vi "Process.vi"(8 "error in (no error)":errorcluster, 11 "SMO.UI":refnum<class "SMO.UI.Template.lvclass">) -> (0 "error out":errorcluster, 3 "SMO.UI out":refnum<class "SMO.UI.Template.lvclass">)   [LabVIEW 2013, in "SMO.UI.Template.lvclass"]
uses:
  SMO.UI.Template.lvclass
  SMO/Typedefs/Parent Call--Enum.ctl
  SMO.UI/SMO.UI.lvclass
  SMO.UI.Template.lvclass/SMO.UI.Template.ctl
  SMO.Template/SMO.Template.lvclass
  SMO/SMO.lvclass
panel:
  in  "OK":bool
  in  "Set Data":bool
  in  "New Data":string
  out "Data":string
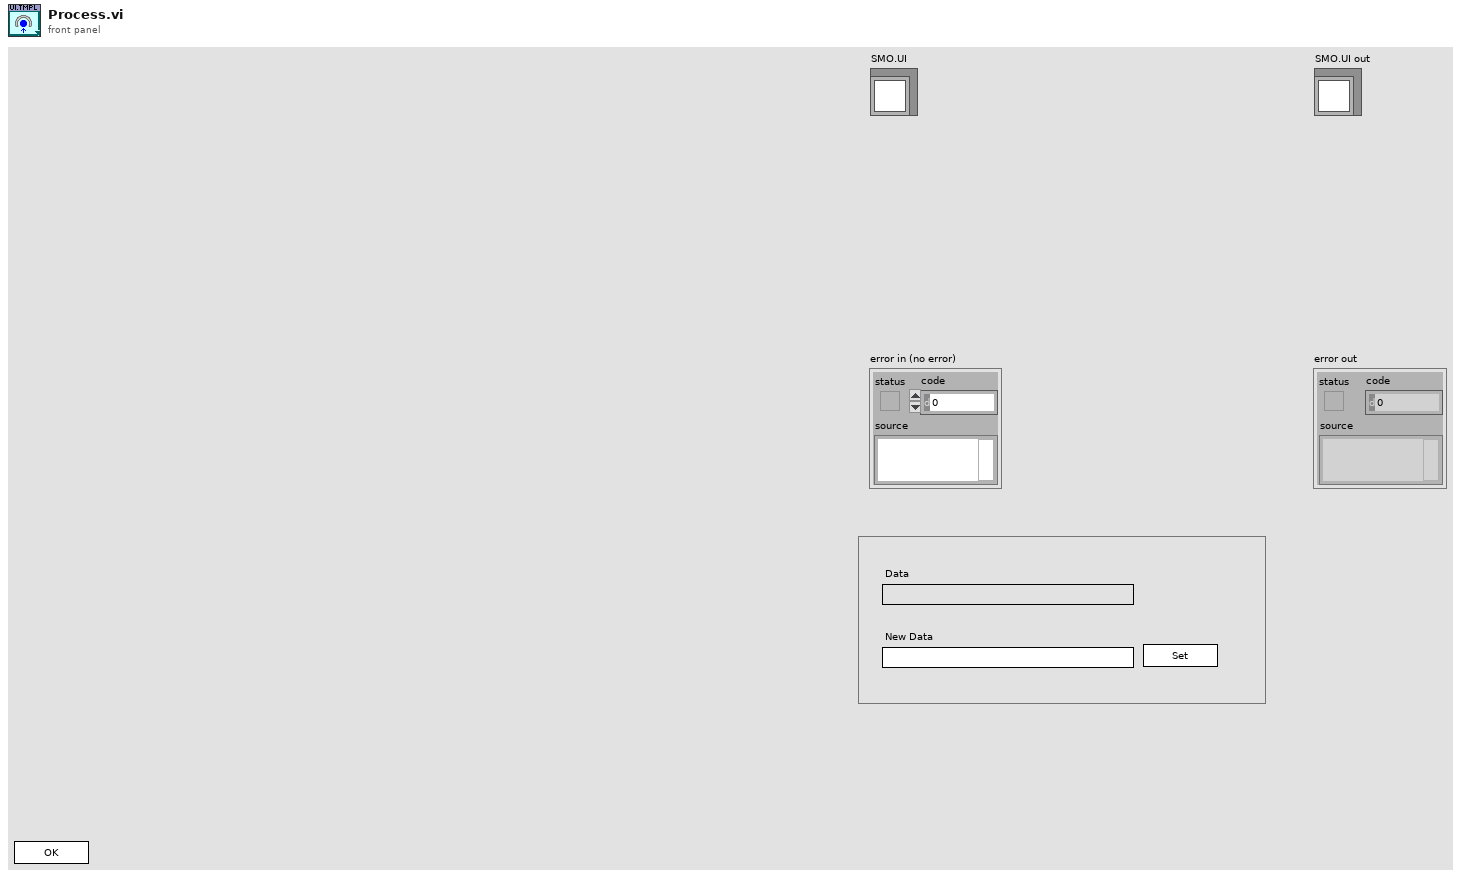
[diagram p1: front panel]
types:
  T1 = typedef "SMO.lvclass/Parent Call--Enum.ctl" = enum16{"Allows parent to run", "Does not request parent to run"}
  T2 = enum32{"invalid app kind", "Development System", "Run Time System", "Student Edition", "Embedded LabVIEW", "Evaluation", "Custom"}
  T3 = enum32{"Invalid", "Standard", "Closed", "Hidden", "Minimized", "Maximized"}
  T4 = cluster{"Core":cluster{"Current VI Reference":refnum<vi>, "Close Panel on Exit?":bool, "error":errorcluster}, "Self Ref":refnum<class "SMO.UI.Template.lvclass">, "Exec.State":enum32{"Bad", "Idle", "Run top level", "Running"}, "SMO.Template":refnum<class "SMO.Template.lvclass">}
  T5 = cluster{"Current VI Reference":refnum<vi>, "Close Panel on Exit?":bool, "error":errorcluster}
  T6 = enum32{"Bad", "Idle", "Run top level", "Running"}
  T7 = typedef "SMO.lvclass/Protected Events.ctl" = cluster{"StopProcesses":refnum<user-event>, "AbortProcesses":refnum<user-event>}
  T8 = cluster{"Event Registration Refnum":refnum<event-registration>, "SMO.UI Public Events":refnum<event-registration>, "SMO.Template Public Events":refnum<event-registration>}
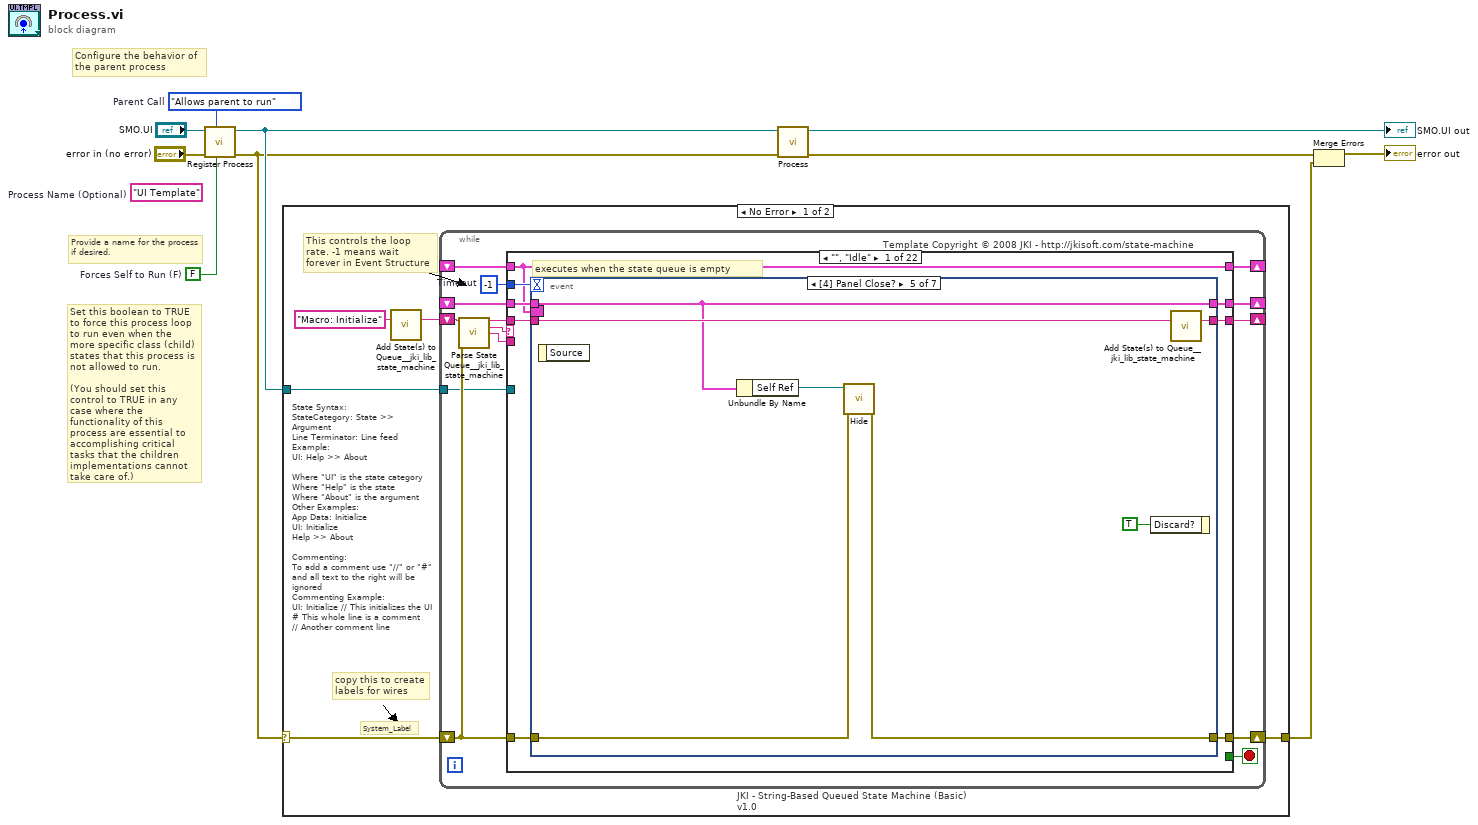
[diagram p0: block diagram]
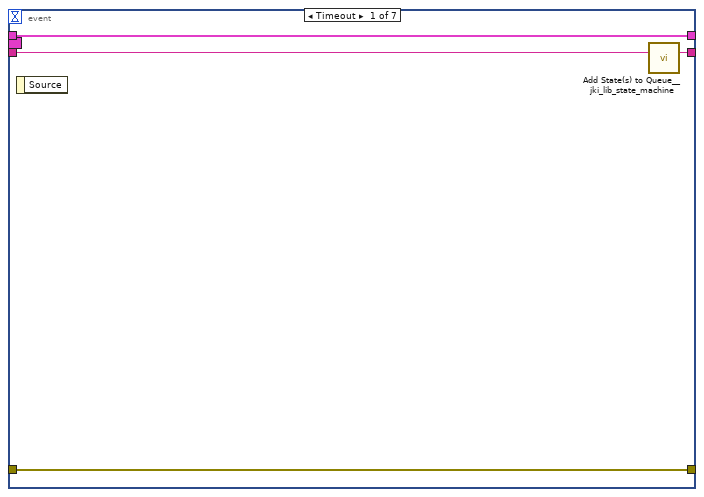
[diagram p2: hidden frame]
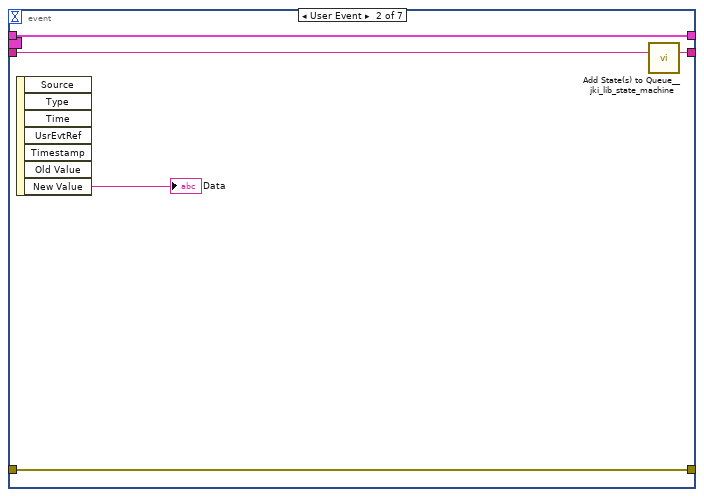
[diagram p3: hidden frame]
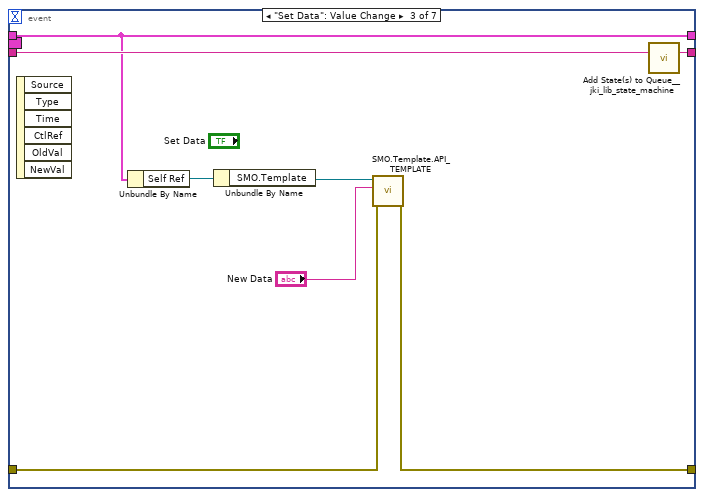
[diagram p4: hidden frame]
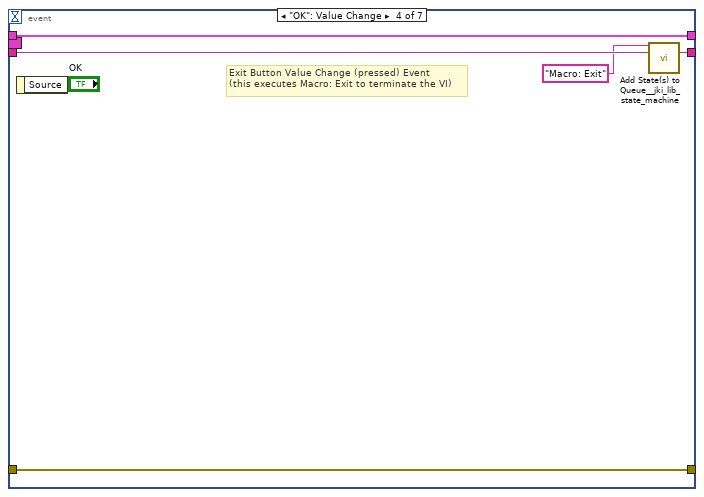
[diagram p5: hidden frame]
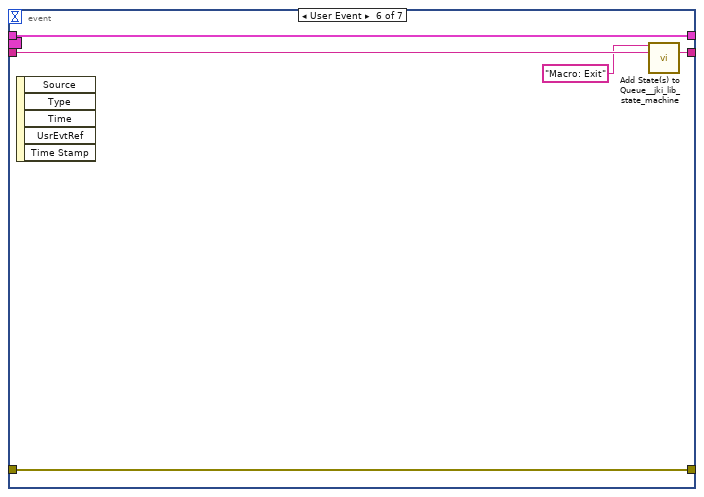
[diagram p6: hidden frame]
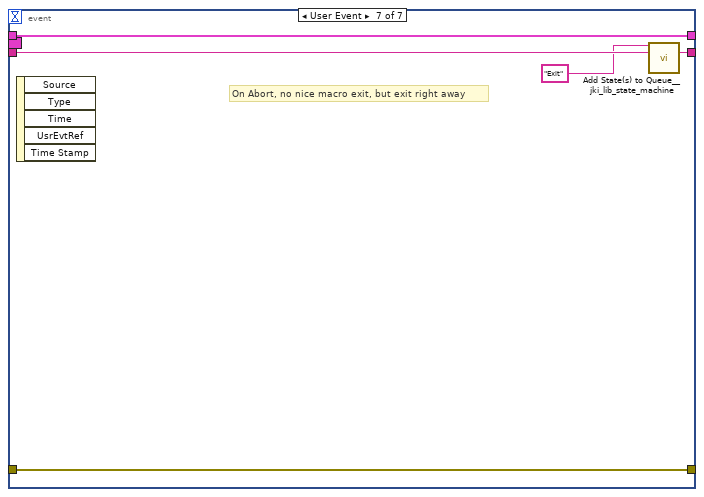
[diagram p7: hidden frame]
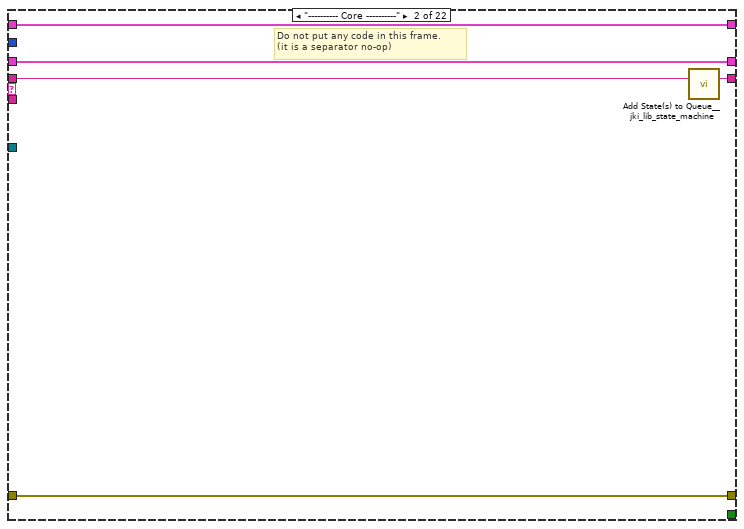
[diagram p8: hidden frame]
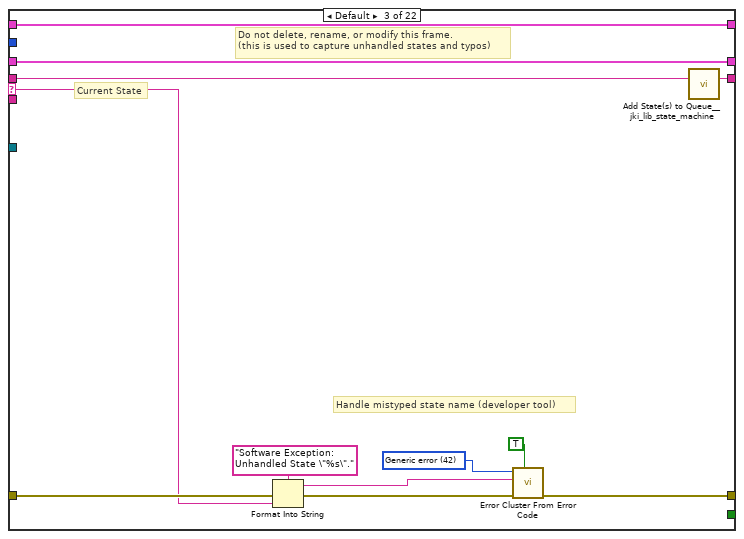
[diagram p9: hidden frame]
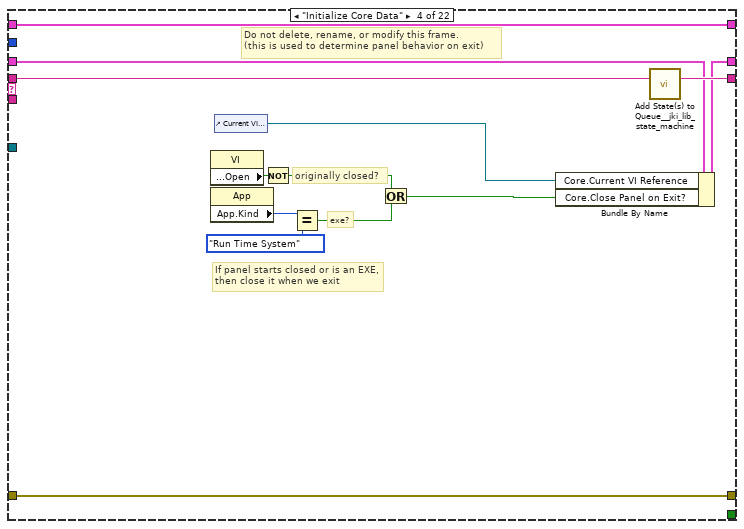
[diagram p10: hidden frame]
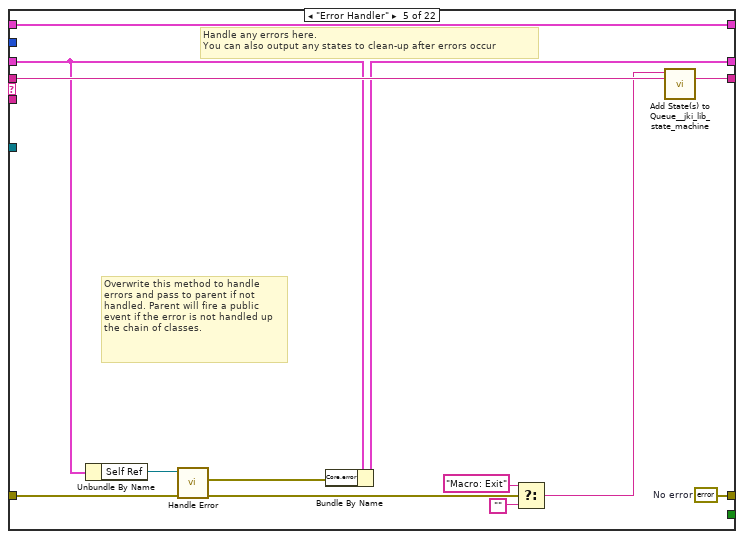
[diagram p11: hidden frame]
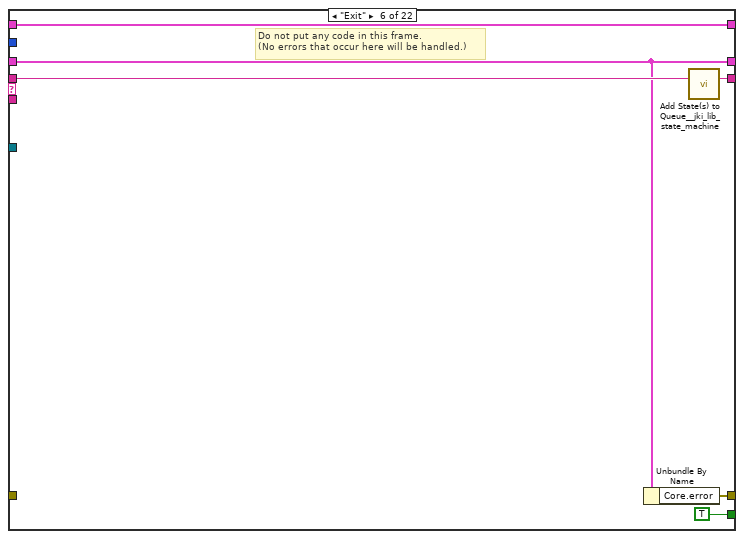
[diagram p12: hidden frame]
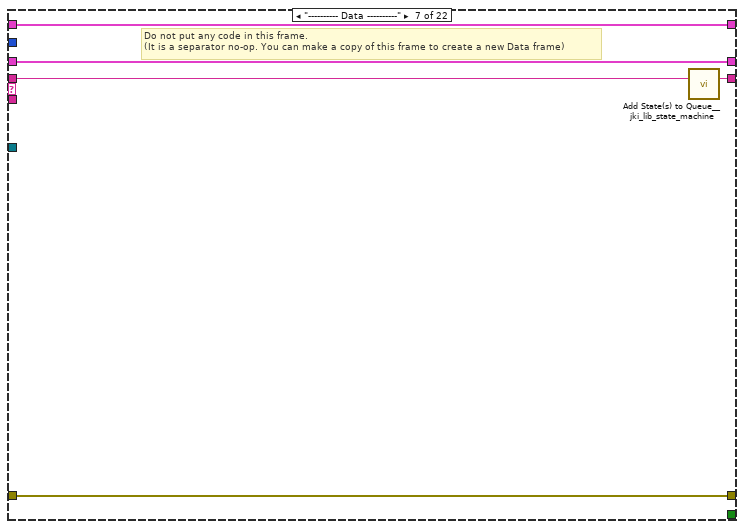
[diagram p13: hidden frame]
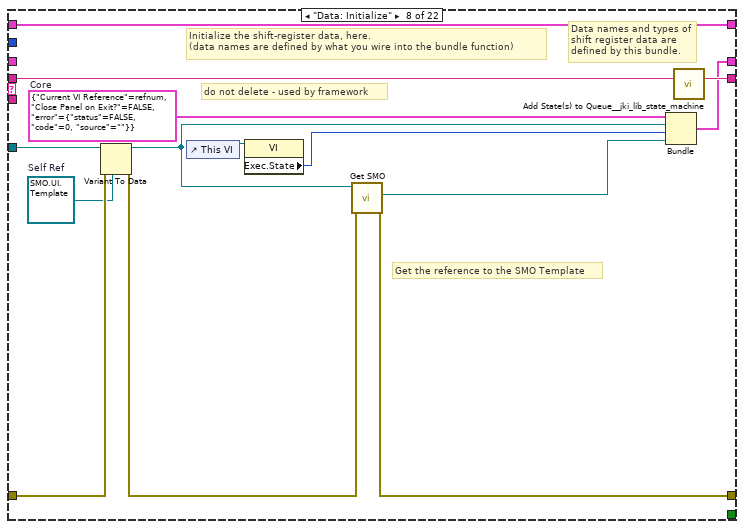
[diagram p14: hidden frame]
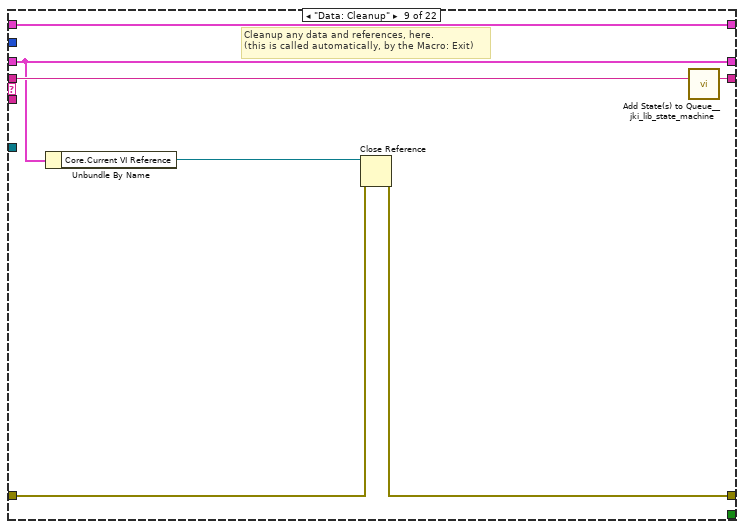
[diagram p15: hidden frame]
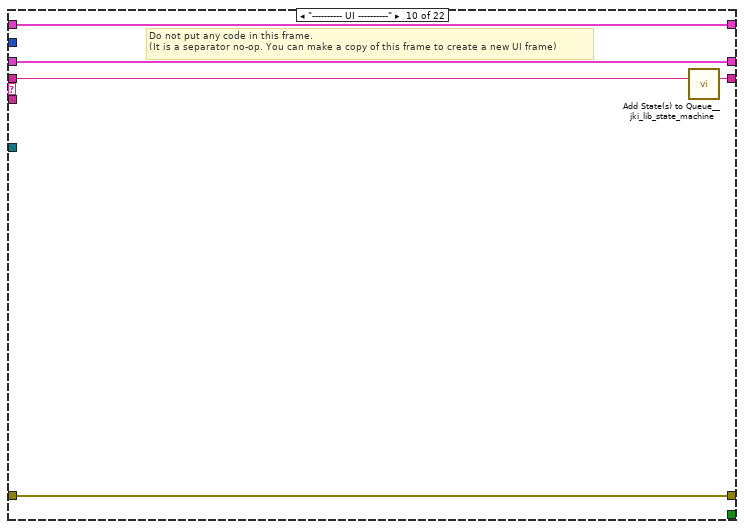
[diagram p16: hidden frame]
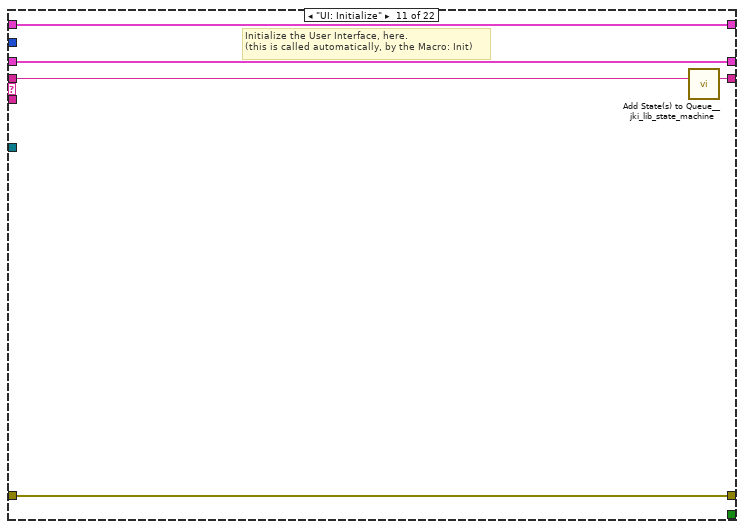
[diagram p17: hidden frame]
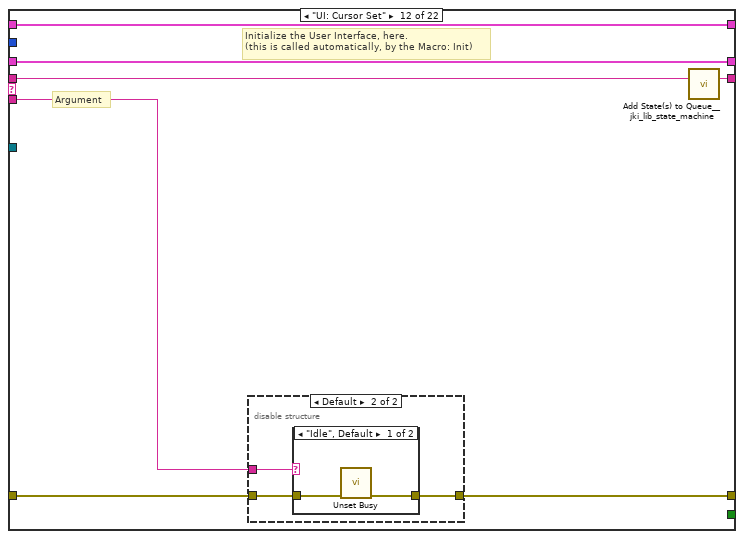
[diagram p18: hidden frame]
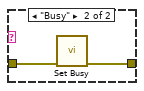
[diagram p20: hidden frame]
diagram:
  w1 = FALSE  # Forces Self to Run (F)
  w2 = Parent_Call--Enum."Allows parent to run"  # Parent Call
  (unwired) "UI Template"  # Process Name (Optional)
  # "Configure the behavior of the parent process"
  # "Provide a name for the process\nif desired."
  # "Set this boolean to TRUE to force this process loop to run even when the more specific class (child) states that this process is not allowed to run.\n\n(You should set this control to TRUE in any case where the functionality of this process are essential to accomplishing critical tasks that the children implementations cannot take care of.)"
  n1 = call "Register Process.vi"("Forces Self to Run (F)"=w1, "Parent Call"=w2, "error in (no error)"="error in (no error)", "SMO"="SMO.UI") -> ("error out"=w4:errorcluster, "SMO out"=w5:refnum<class "SMO.UI.Template.lvclass">)  [unwired: 6 in]
  n2 = case shown="No Error" w4 {
    selector: w4 -> [w12 w294]
    tunnel: w5 -> [w13 _]
    tunnel: [w11 w294] -> w3
    frame No Error {
      # "State Syntax:\nStateCategory: State >> Argument\nLine Terminator: Line feed\nExample:\nUI: Help >> About\n\nWhere \"UI\" is the state category\nWhere \"Help\" is the state\nWhere \"About\" is the argument\nOther Examples:\nApp Data: Initialize\nUI: Initialize\nHelp >> About\n\nCommenting:\nTo add a comment use \"//\" or \"#\" and all text to the right will be ignored\nCommenting Example:\nUI: Initialize // This initializes the UI\n# This whole line is a comment\n// Another comment line"
      # "copy this to create labels for wires"
      # "This controls the loop rate. -1 means wait forever in Event Structure"
      # "System_Label"
      n3 = call <vilib>:"Add State(s) to Queue__jki_lib_state_machine.vi"("State(s) in (\"\")"="Macro: Initialize") -> ("States Out"=w15:string)  [unwired: 14 in]
      n4 = while "JKI - String-Based Queued State Machine (Basic) v1.0" {
        shift-right: [w22] -> _
        shift-left: _ -> [w21]
        shift-right: [w25] -> w11
        shift-left: w12 -> [w19]
        shift-right: [w24] -> _
        shift-left: w15 -> [w26]
        tunnel: w13 -> [w18]
        shift-right: [w17] -> _
        shift-left: _ -> [w16]
        stop <- w23 stop-if-true
        w20 = -1  # Timeout
        # "Template Copyright © 2008 JKI - http://jkisoft.com/state-machine"
        n5 = call <vilib>:"Parse State Queue__jki_lib_state_machine.vi"("State Queue"=w26, "Error In (no error)"=w19) -> ("Remaining States"=w28:string, "Current State"=w29:string, "Arguments"=w27:string)  [unwired: 11 in]
        n6 = case shown="\"\", \"Idle\"" w29 {
          selector: w29 -> [_ _ w83 _ _ _ _ _ _ _ _ _ _ _ _ _ _ _ _ _ _ _]
          tunnel: w28 -> [w37 w81 w87 w106 w119 w125 w130 w144 w151 w156 w161 w168 w184 w216 w225 w239 w244 w255 w265 w282 w288 w293]
          tunnel: w27 -> [_ _ _ _ _ _ _ _ _ _ _ w162 w178 _ _ _ _ _ _ _ _ _]
          tunnel: w21 -> [w35 w78 w85 w97 w110 w121 w127 _ w146 w153 w159 w166 w180 w213 w221 w230 w241 w251 w262 w280 w286 w290]
          tunnel: [w34 w79 w89 w103 w107 w120 w128 w132 w147 w154 w158 w163 w181 w214 w223 w237 w242 w252 w263 w266 w283 w291] -> w25
          tunnel: w19 -> [w33 w79 w88 w103 w111 _ w128 w141 w148 w154 w158 w164 w182 w214 w223 w237 w242 w248 w263 w271 w284 w291]
          tunnel: [w36 w80 w86 w105 w118 w124 w129 w143 w150 w155 w160 w167 w183 w215 w224 w238 w243 w254 w264 w281 w287 w292] -> w24
          tunnel: [_ _ _ _ _ TRUE _ _ _ _ _ _ _ _ _ _ _ _ _ _ _ _] -> w23
          tunnel: [w32 w78 w85 w104 w109 w121 w127 w142 w146 w153 w159 w166 w180 w213 w221 w230 w241 w251 w262 w280 w286 w290] -> w22
          tunnel: w20 -> [w31 _ _ _ _ _ _ _ _ _ _ _ _ _ _ _ _ _ _ _ _ _]
          tunnel: w18 -> [_ _ _ _ _ _ _ w140 _ _ _ _ _ _ _ _ _ _ _ _ _ _]
          tunnel: [w30 w77 w82 w94 w117 w122 w126 w139 w145 w152 w157 w165 w177 w212 w222 w231 w240 w253 w261 w274 w285 w289] -> w17
          tunnel: w16 -> [w30 w77 w82 w94 w117 w122 w126 w139 w145 w152 w157 w165 w177 w212 w222 w231 w240 w253 w261 _ w285 w289]
          frame "", "Idle" {
            # "executes when the state queue is empty"
            n7 = event shown="[4] Panel Close?" {
              selector: w30 -> [_ _ _ _ _ _ _]
              dyn-events: _ -> [_ _ _ _ _ _ _]
              timeout: w31 -> [_ _ _ _ _ _ _]
              tunnel: w37 -> [w41 w46 w54 w59 w66 w71 w76]
              tunnel: [w40 w45 w53 w58 w65 w70 w75] -> w36
              tunnel: w35 -> [w38 w43 w49 w56 w63 w68 w73]
              tunnel: [w39 w44 w47 w57 w60 w69 w74] -> w34
              tunnel: w33 -> [w39 w44 w48 w57 w61 w69 w74]
              tunnel: [w38 w43 w49 w56 w63 w68 w73] -> w32
              event Timeout {
                n8 = event-data() -> ()  [unwired: 1 in, 1 out]
                n9 = call <vilib>:"Add State(s) to Queue__jki_lib_state_machine.vi"("State(s) in (\"\")"=w41) -> ("States Out"=w40:string)  [unwired: 14 in]
              }
              event User Event {
                n10 = event-data() -> ("New Value"=→"Data":string)  [unwired: 1 in, 6 out]
                n11 = call <vilib>:"Add State(s) to Queue__jki_lib_state_machine.vi"("State(s) in (\"\")"=w46) -> ("States Out"=w45:string)  [unwired: 14 in]
              }
              event "Set Data": Value Change {
                n12 = event-data() -> ()  [unwired: 1 in, 6 out]
                n13 = Unbundle By Name(w49) -> ("Self Ref"=w52:refnum<class "SMO.UI.Template.lvclass">)
                n14 = Unbundle By Name(w52) -> ("SMO.Template"=w51:refnum<class "SMO.Template.lvclass">)
                n15 = call "SMO.Template.API_TEMPLATE.vi"("error in (no error)"=w48, "myData"="New Data", "SMO"=w51) -> ("error out"=w47:errorcluster)  [unwired: 6 in, 2 out]
                n16 = call <vilib>:"Add State(s) to Queue__jki_lib_state_machine.vi"("State(s) in (\"\")"=w54) -> ("States Out"=w53:string)  [unwired: 14 in]
              }
              event "OK": Value Change {
                # "Exit Button Value Change (pressed) Event\n(this executes Macro: Exit to terminate the VI)"
                n17 = event-data() -> ()  [unwired: 1 in, 1 out]
                n18 = call <vilib>:"Add State(s) to Queue__jki_lib_state_machine.vi"("State(s) in Front (\"\")"="Macro: Exit", "State(s) in (\"\")"=w59) -> ("States Out"=w58:string)  [unwired: 13 in]
              }
              event Panel Close? {
                n19 = event-data() -> ()  [unwired: 1 in, 1 out]
                n20 = Unbundle By Name(w63) -> ("Self Ref"=w62:refnum<class "SMO.UI.Template.lvclass">)
                n21 = call "Hide.vi"("error in (no error)"=w61, "SMO.UI"=w62) -> ("error out"=w60:errorcluster)  [unwired: 8 in, 1 out]
                n22 = event-data("Discard?"=TRUE) -> ()  [unwired: 1 in, 1 out]
                n23 = call <vilib>:"Add State(s) to Queue__jki_lib_state_machine.vi"("State(s) in (\"\")"=w66) -> ("States Out"=w65:string)  [unwired: 14 in]
              }
              event User Event {
                n24 = event-data() -> ()  [unwired: 1 in, 5 out]
                n25 = call <vilib>:"Add State(s) to Queue__jki_lib_state_machine.vi"("State(s) in Front (\"\")"="Macro: Exit", "State(s) in (\"\")"=w71) -> ("States Out"=w70:string)  [unwired: 13 in]
              }
              event User Event {
                # "On Abort, no nice macro exit, but exit right away"
                n26 = event-data() -> ()  [unwired: 1 in, 5 out]
                n27 = call <vilib>:"Add State(s) to Queue__jki_lib_state_machine.vi"("State(s) in Front (\"\")"="Exit", "State(s) in (\"\")"=w76) -> ("States Out"=w75:string)  [unwired: 13 in]
              }
            }
          }
          frame "---------- Core ----------" {
            # "Do not put any code in this frame.\n(it is a separator no-op)"
            n28 = call <vilib>:"Add State(s) to Queue__jki_lib_state_machine.vi"("State(s) in (\"\")"=w81) -> ("States Out"=w80:string)  [unwired: 14 in]
          }
          frame Default {
            w92 = 42 items=["No error", "Argument error", "Memory is full", "Out of zone", "End of file", "File already open", "Generic file I/O error", "File not found", "File permission error", "Disk is full", "Duplicate path", "Too many files open", "System feature not enabled", "Resource file not found", "Cannot add resource", "Resource not found", "Image not found", "Image memory error", "Pen does not exist", "Config type invalid", "Config token not found", "Config parse error", "Config memory error", "Bad external code format", "Bad external code offset", "External code not present", "Null window", "Destroy window error", "Null menu", "Print aborted", "Bad print record", "Print driver error", "Windows error during printing", "Memory error during printing", "Print dialog error", "Generic print error", "Invalid device refnum", "Device not found", "Device parameter error", "Device unit error", "Cannot open device", "Device call aborted", "Generic error", "Cancelled by user", "Object ID too low", "Object ID too high", "Object not in heap", "Unknown heap", "Unknown object (invalid DefProc)", "Unknown object (DefProc not in table)", "Message out of range", "Invalid (null) method", "Unknown message", "Manager call not supported", "Bad address", "Network operation in progress", "Network operation timed out", "Connection is busy", "Network attribute not supported", "Network error", "Address in use", "System out of memory", "Connection aborted", "Connection refused", "Not connected", "Already connected", "Connection closed", "Initialization error (interapplication manager)", "Bad occurrence", "Wait on unbound occurrence handler", "Occurrence queue overflow", "Datalog type conflict", "Unused", "Unrecognized type (interapplication manager)", "Memory corrupt", "Failed to make temporary DLL", "Old CIN version", "Drag socket not found", "Failed to load drop-object", "Failed to register OLE object", "Failed to release OLE object", "Format specifier type mismatch", "Unknown format specifier", "Too few format specifiers", "Too many format specifiers", "Scan failed", "Newer CIN version", "Error converting to variant", "Runtime menu error", "Password tampered", "Variant attribute not found", "Incompatible variant data type", "Event data is not available", "Event Store is not present", "Occurrence is not found", "Event Queue is not created", "Event info is not available", "Refnum passed is NULL", "Error retrieving Class GUID", "Error retrieving CoClass GUID", "Error retrieving TypeLib GUID.", "Bad built application magic bytes.", "Specific driver is different from the specific driver associated with the Logical Name.", "There is no session opened to the class driver.", "Max Error", "MAX - Error with config objects", "MAX - Error loading configuration", "MAX - Group not supported"]
            # "Current State"
            # "Do not delete, rename, or modify this frame.\n(this is used to capture unhandled states and typos)"
            # "Handle mistyped state name (developer tool)"
            n29 = Format Into String(format string="Software Exception: Unhandled State \"%s\"." ("message"), error in=w88, w83) -> (resulting string=w91:string, error out=w90:errorcluster)  [unwired: 1 in]
            n30 = call <vilib>:"Error Cluster From Error Code.vi"("show call chain? (False)"=TRUE, "error in (no error)"=w90, "error message (\"\")"=w91, "error code (0)"=w92) -> ("error out"=w89:errorcluster)  [unwired: 5 in]
            n31 = call <vilib>:"Add State(s) to Queue__jki_lib_state_machine.vi"("State(s) in (\"\")"=w87) -> ("States Out"=w86:string)  [unwired: 14 in]
          }
          frame "Initialize Core Data" {
            # "Do not delete, rename, or modify this frame.\n(this is used to determine panel behavior on exit)"
            # "originally closed?"
            # "exe?"
            # "If panel starts closed or is an EXE, then close it when we exit"
            n32 = property class="VI"() -> ("Front Panel.Open"=w102:bool)  [unwired: 2 in, 2 out]
            n33 = property class="App"() -> ("App.Kind"=w101:T2)  [unwired: 2 in, 2 out]
            n34 = control-ref of="Current VI Reference"() -> (w95:refnum<vi>)
            n35 = Not(x=w102) -> (.not. x?=w99:bool)
            n36 = Equal?(x=w101, y=T2."Run Time System" ("Application:Kind")) -> (x = y?=w98:bool)
            n37 = Or(x=w99, y=w98) -> (x .or. y?=w96:bool)
            n38 = Bundle By Name(cluster=w97, "Core.Current VI Reference"=w95, "Core.Close Panel on Exit?"=w96) -> (w104:T4)
            n39 = call <vilib>:"Add State(s) to Queue__jki_lib_state_machine.vi"("State(s) in (\"\")"=w106) -> ("States Out"=w105:string)  [unwired: 14 in]
          }
          frame "Error Handler" {
            w107 = errorcluster {"status"=FALSE, "code"=0, "source"=""}  # No error
            # "Overwrite this method to handle errors and pass to parent if not handled. Parent will fire a public event if the error is not handled up the chain of classes."
            # "Handle any errors here.\nYou can also output any states to clean-up after errors occur"
            n40 = Unbundle By Name(w110) -> ("Self Ref"=w112:refnum<class "SMO.UI.Template.lvclass">)
            n41 = call-dynamic "Handle Error.vi"("error in"=w111, "SMO"=w112) -> ("handling error"=w115:errorcluster, "Unhandled error"=w116:errorcluster)  [unwired: 7 in, 1 out]
            n42 = Bundle By Name(cluster=w110, "Core.error"=w116) -> (w109:T4)
            n43 = Select(t="Macro: Exit", s=w115, f="") -> (s? t:f=w108:string)
            n44 = call <vilib>:"Add State(s) to Queue__jki_lib_state_machine.vi"("State(s) in Front (\"\")"=w108, "State(s) in (\"\")"=w119) -> ("States Out"=w118:string)  [unwired: 13 in]
          }
          frame "Exit" {
            # "Do not put any code in this frame.\n(No errors that occur here will be handled.)"
            n45 = Unbundle By Name(w121) -> ("Core.error"=w120:errorcluster)
            n46 = call <vilib>:"Add State(s) to Queue__jki_lib_state_machine.vi"("State(s) in (\"\")"=w125) -> ("States Out"=w124:string)  [unwired: 14 in]
          }
          frame "---------- Data ----------" {
            # "Do not put any code in this frame.\n(It is a separator no-op. You can make a copy of this frame to create a new Data frame)"
            n47 = call <vilib>:"Add State(s) to Queue__jki_lib_state_machine.vi"("State(s) in (\"\")"=w130) -> ("States Out"=w129:string)  [unwired: 14 in]
          }
          frame "Data: Initialize" {
            w131 = T5 {"Current VI Reference"=refnum, "Close Panel on Exit?"=FALSE, "error"={"status"=FALSE, "code"=0, "source"=""}}  # Core
            w136 = refnum<class "SMO.UI.Template.lvclass"> refnum  # Self Ref
            # "Get the reference to the SMO Template"
            # "do not delete - used by framework"
            # "Data names and types of shift register data are defined by this bundle."
            # "Initialize the shift-register data, here.\n(data names are defined by what you wire into the bundle function)"
            n48 = Variant To Data(error in=w141, type=w136, Variant=w140) -> (data=w135:refnum<class "SMO.UI.Template.lvclass">, error out=w133:errorcluster)
            n49 = control-ref of="This VI"() -> (w137:refnum<vi>)
            n50 = property class="VI"(reference=w137) -> ("Exec.State"=w138:T6)  [unwired: 1 in, 2 out]
            n51 = call "Get SMO.vi"("error in (no error)"=w133, "SMO.UI"=w135) -> ("error out"=w132:errorcluster, "SMO.Template"=w134:refnum<class "SMO.Template.lvclass">)  [unwired: 7 in, 1 out]
            n52 = Bundle("Core"=w131, "Self Ref"=w135, "Exec.State"=w138, "SMO.Template"=w134) -> (w142:T4)  [unwired: 1 in]
            n53 = call <vilib>:"Add State(s) to Queue__jki_lib_state_machine.vi"("State(s) in (\"\")"=w144) -> ("States Out"=w143:string)  [unwired: 14 in]
          }
          frame "Data: Cleanup" {
            # "Cleanup any data and references, here.\n(this is called automatically, by the Macro: Exit)"
            n54 = Unbundle By Name(w146) -> ("Core.Current VI Reference"=w149:refnum<vi>)
            n55 = Close Reference(reference=w149, error in (no error)=w148) -> (error out=w147:errorcluster)
            n56 = call <vilib>:"Add State(s) to Queue__jki_lib_state_machine.vi"("State(s) in (\"\")"=w151) -> ("States Out"=w150:string)  [unwired: 14 in]
          }
          frame "---------- UI ----------" {
            # "Do not put any code in this frame.\n(It is a separator no-op. You can make a copy of this frame to create a new UI frame)"
            n57 = call <vilib>:"Add State(s) to Queue__jki_lib_state_machine.vi"("State(s) in (\"\")"=w156) -> ("States Out"=w155:string)  [unwired: 14 in]
          }
          frame "UI: Initialize" {
            # "Initialize the User Interface, here.\n(this is called automatically, by the Macro: Init)"
            n58 = call <vilib>:"Add State(s) to Queue__jki_lib_state_machine.vi"("State(s) in (\"\")"=w161) -> ("States Out"=w160:string)  [unwired: 14 in]
          }
          frame "UI: Cursor Set" {
            # "Argument"
            # "Initialize the User Interface, here.\n(this is called automatically, by the Macro: Init)"
            n59 = disable-structure shown="Default" {
              disable-tunnel: w164 -> [w169 w172]
              disable-tunnel: [w169 w171] -> w163
              disable-tunnel: w162 -> [_ w170]
              frame condition #0 {
              }
              frame condition #1 (active) {
                n60 = case shown="\"Idle\", Default" w170 {
                  tunnel: w172 -> [w174 w176]
                  tunnel: [w173 w175] -> w171
                  frame "Idle", Default {
                    n61 = call <vilib>:"Unset Busy.vi"("error in (no error)"=w174) -> ("error out"=w173:errorcluster)  [unwired: 10 in]
                  }
                  frame "Busy" {
                    n62 = call <vilib>:"Set Busy.vi"("error in (no error)"=w176) -> ("error out"=w175:errorcluster)  [unwired: 9 in, 1 out]
                  }
                }
              }
            }
            n63 = call <vilib>:"Add State(s) to Queue__jki_lib_state_machine.vi"("State(s) in (\"\")"=w168) -> ("States Out"=w167:string)  [unwired: 14 in]
          }
          frame "UI: Front Panel State" {
            # "Argument"
            # "Set Front Panel Open or Closed\n(Usage: \"UI: Front Panel State >> Open|Close\")"
            n64 = Unbundle By Name(w180) -> ("Core.Current VI Reference"=w179:refnum<vi>)
            n65 = disable-structure shown="Default" {
              disable-tunnel: w182 -> [w188 w211]
              disable-tunnel: [w187 w211] -> w181
              disable-tunnel: w179 -> [w186 _]
              disable-tunnel: w178 -> [w185 _]
              frame condition #0 (active) {
                n66 = case shown="\"Open\", Default" w185 {
                  tunnel: w188 -> [w192 w205]
                  tunnel: [w194 w206] -> w187
                  tunnel: w186 -> [w193 w203]
                  frame "Open", Default {
                    n67 = property class="VI"(reference=w193, error in=w192) -> (reference out=w190:refnum<vi>, error out=w191:errorcluster, "Front Panel.Open"=w189:bool)
                    n68 = case shown="False" w189 {
                      tunnel: [w197 w200] -> w194
                      tunnel: w191 -> [w196 w200]
                      tunnel: w190 -> [w195 _]
                      frame False {
                        n69 = invoke class="VI" method="FP.Open"(reference=w195, error in=w196, "Activate"=TRUE, "State"=T3."Standard") -> (error out=w197:errorcluster)  [unwired: 1 in, 4 out]
                      }
                      frame True {
                      }
                    }
                  }
                  frame "Close" {
                    n70 = property class="VI"(reference=w203, error in=w205) -> (reference out=w202:refnum<vi>, error out=w204:errorcluster, "Front Panel.Open"=w201:bool)
                    n71 = case shown="True" w201 {
                      tunnel: [w207 w210] -> w206
                      tunnel: w204 -> [w207 w209]
                      tunnel: w202 -> [_ w208]
                      frame False {
                      }
                      frame True {
                        n72 = invoke class="VI" method="FP.Close"(reference=w208, error in=w209) -> (error out=w210:errorcluster)  [unwired: 1 in, 2 out]
                      }
                    }
                  }
                }
              }
              frame condition #1 {
              }
            }
            n73 = call <vilib>:"Add State(s) to Queue__jki_lib_state_machine.vi"("State(s) in (\"\")"=w184) -> ("States Out"=w183:string)  [unwired: 14 in]
          }
          frame "---------- Macro ----------" {
            # "Do not put any code in this frame.\n(It is a separator no-op. You can make a copy of this frame to create a new Macro frame)"
            n74 = call <vilib>:"Add State(s) to Queue__jki_lib_state_machine.vi"("State(s) in (\"\")"=w216) -> ("States Out"=w215:string)  [unwired: 14 in]
          }
          frame "Macro: Initialize" {
            w219 = "UI: Initialize\n//UI: Front Panel State >> Open"  # UI: Initialize //UI: Front Panel State >> Open
            # "Initialization Macro\n(This is called once, when the VI starts)"
            n75 = call <vilib>:"Add State(s) to Queue__jki_lib_state_machine.vi"("State(s) in Front (\"\")"="Data: Initialize\nInitialize Core Data\nEvents: Register", "State(s) in (\"\")"="Process: Sync", "State(s) at Back (\"\")"=w219) -> ("States Out"=w218:string)  [unwired: 12 in]
            n76 = call <vilib>:"Add State(s) to Queue__jki_lib_state_machine.vi"("State(s) in Front (\"\")"=w218, "State(s) in (\"\")"=w225) -> ("States Out"=w224:string)  [unwired: 13 in]
          }
          frame "Macro: Exit" {
            # "Exit Macro\n(This is called once, when the VI exits)"
            n77 = Unbundle By Name(w230) -> ("Core.Close Panel on Exit?"=w236:bool)
            n78 = Select(t="UI: Front Panel State >> Close", s=w236, f="") -> (s? t:f=w233:string)
            n79 = call <vilib>:"Add State(s) to Queue__jki_lib_state_machine.vi"("State(s) in Front (\"\")"="Data: Cleanup\nEvents: Unregister", "State(s) in (\"\")"="Process: Sync", "State(s) at Back (\"\")"="Exit") -> ("States Out"=w227:string)  [unwired: 12 in]
            n80 = call <vilib>:"Add State(s) to Queue__jki_lib_state_machine.vi"("State(s) in (\"\")"=w233, "State(s) at Back (\"\")"=w227) -> ("States Out"=w232:string)  [unwired: 13 in]
            n81 = call <vilib>:"Add State(s) to Queue__jki_lib_state_machine.vi"("State(s) in Front (\"\")"=w232, "State(s) in (\"\")"=w239) -> ("States Out"=w238:string)  [unwired: 13 in]
          }
          frame "---------- Process ----------" {
            # "Template Separator\n(You can make a copy of, or modify, this frame)"
            n82 = call <vilib>:"Add State(s) to Queue__jki_lib_state_machine.vi"("State(s) in (\"\")"=w244) -> ("States Out"=w243:string)  [unwired: 14 in]
          }
          frame "Process: Sync" {
            # "Template Separator\n(You can make a copy of, or modify, this frame)"
            n83 = Unbundle By Name(w251) -> ("Self Ref"=w250:refnum<class "SMO.UI.Template.lvclass">)
            n84 = call "isProcessAllowedRun.vi"("error in (no error)"=w248, "SMO in"=w250) -> ("error out"=w247:errorcluster, "Run Allowed"=w246:bool, "SMO out"=w249:refnum<class "SMO.UI.Template.lvclass">)  [unwired: 7 in]
            n85 = case shown="True" w246 {
              tunnel: [w257 w260] -> w252
              tunnel: w249 -> [_ w259]
              tunnel: w247 -> [w257 w258]
              tunnel: ["Macro: Exit" _] -> w245
              frame False {
              }
              frame True {
                n86 = call "WaitOnProcessSync.vi"("error in (no error)"=w258, "SMO"=w259) -> ("error out"=w260:errorcluster)  [unwired: 8 in, 1 out]
              }
            }
            n87 = call <vilib>:"Add State(s) to Queue__jki_lib_state_machine.vi"("State(s) in Front (\"\")"=w245, "State(s) in (\"\")"=w255) -> ("States Out"=w254:string)  [unwired: 13 in]
          }
          frame "---------- Events ----------" {
            # "Template Separator\n(You can make a copy of, or modify, this frame)"
            n88 = call <vilib>:"Add State(s) to Queue__jki_lib_state_machine.vi"("State(s) in (\"\")"=w265) -> ("States Out"=w264:string)  [unwired: 14 in]
          }
          frame "Events: Register" {
            # "Base Class Protected Events"
            # "Your code here.\n(You can make a copy of, or modify, this frame)"
            n89 = Unbundle By Name(w280) -> ("Self Ref"=w278:refnum<class "SMO.UI.Template.lvclass">, "SMO.Template"=w277:refnum<class "SMO.Template.lvclass">)
            n90 = call "GetProtectedEvents.vi"("SMO"=w278) -> ("error out"=w267:errorcluster, "SMO Protected Events"=w279:T7, "SMO out"=w273:refnum<class "SMO.UI.Template.lvclass">)  [unwired: 8 in]
            n91 = call "SMO.UI.GetPublicEventsRegistration.vi"("SMO.UI"=w273) -> ("error out"=w268:errorcluster, "SMO.UI Public Events"=w272:refnum<event-registration>)  [unwired: 8 in, 1 out]
            n92 = call "SMO.Template.GetPublicEventsRegistration.vi"("SMO"=w277) -> ("error out"=w269:errorcluster, "SMO.Template Public Events"=w276:refnum<event-registration>)  [unwired: 8 in, 1 out]
            n93 = register-events(w279) -> (reference out=w275:refnum<event-registration>, error out=w270:errorcluster)  [unwired: 2 in]
            n94 = Merge Errors(w270, w269, w268, w267, w271) -> (w266:errorcluster)
            n95 = Bundle("Event Registration Refnum"=w275, "SMO.UI Public Events"=w272, "SMO.Template Public Events"=w276) -> (w274:T8)  [unwired: 1 in]
            n96 = call <vilib>:"Add State(s) to Queue__jki_lib_state_machine.vi"("State(s) in (\"\")"=w282) -> ("States Out"=w281:string)  [unwired: 14 in]
          }
          frame "Events: Unregister" {
            n97 = Unregister For Events(event registration refnum=w285, error in=w284) -> (error out=w283:errorcluster)
            n98 = call <vilib>:"Add State(s) to Queue__jki_lib_state_machine.vi"("State(s) in (\"\")"=w288) -> ("States Out"=w287:string)  [unwired: 14 in]
          }
          frame "---------MsgAction---------" {
            # "MsgAction Separator\n(You can make a copy of, or modify, this frame)"
            n99 = call <vilib>:"Add State(s) to Queue__jki_lib_state_machine.vi"("State(s) in (\"\")"=w293) -> ("States Out"=w292:string)  [unwired: 14 in]
          }
        }
      }
    }
    frame Error {
    }
  }
  n100 = call-parent "Process.vi"("error in (no error)"=w4, "SMO.UI"=w5) -> ("error out"=w10:errorcluster, "SMO.UI out"=→"SMO.UI out":refnum<class "SMO.UI.Template.lvclass">)  [unwired: 8 in]
  n101 = Merge Errors(w10, w3) -> (→"error out":errorcluster)
